vi "Handle Command.vi"(8 "error in":errorcluster, 10 "Change iSpkEn in":refnum<class "Change iSpk Signal.lvclass">, 11 "Object In":refnum<class>) -> (0 "error out":errorcluster, 1 "Command Successful?":bool, 2 "Change iSpkEn out":refnum<class "Change iSpk Signal.lvclass">, 3 "Object Out":refnum<class>)   [LabVIEW 2018, in "ePAS Library.lvlib" / "Change iSpk Signal.lvclass"]
doc: "Abstract method for accomplishing the execution of a command directed to an instrument object on the wire."
uses:
  Change iSpk Signal.lvclass
  Instrument/ePAS.lvclass
  C:/Users/Labview/Documents/exscalabar_server/reusable/Instrument/Instrument.lvclass
  Instrument/ePAS.lvclass/ePAS.ctl
  Change iSpk Signal.lvclass/Change iSpk Signal.ctl
  reusable/Instrument/Instrument.lvclass/Instrument.ctl
  reusable/Instrument/Read ExtCom.vi
  reusable/Instrument/Read Log Session.vi
  <vilib>/Utility/error.llb/Error Cluster From Error Code.vi
  <vilib>/rvi/errors/niLvFpgaAdjustHostInterfaceError.vi
  <userlib>/_Session Fwk/Session - Root.lvclass
  <vilib>/rvi/interface/nirviReadWriteControl/nirviReadWriteControl.xnode
  FPGA/R FPGA Ref.ctl
  FPGA Bitfiles/FPGAServer.lvbitx
  FPGA/Session/Exscalabar FPGA.lvclass
  ePAS Library.lvlib
  reusable/Session APIs/Session Log/System Log.lvclass
  NiFpgaLv.dll
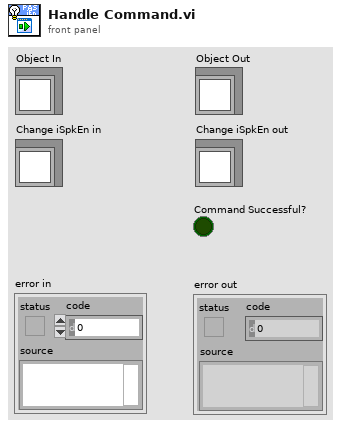
[diagram p1: front panel]
types:
  T1 = typedef "Session - Root.lvclass/Session Handle.ctl" = refnum<data-value>
  T2 = typedef "ePAS Library.lvlib/R FPGA Ref.ctl" = refnum<k20>
  T3 = cluster{"iSpkEn[0]":bool, "iSpkEn[1]":bool, "iSpkEn[2]":bool, "iSpkEn[3]":bool, "iSpkEn[4]":bool}
  T4 = cluster{"tag":string, "section":string, "data":variant}
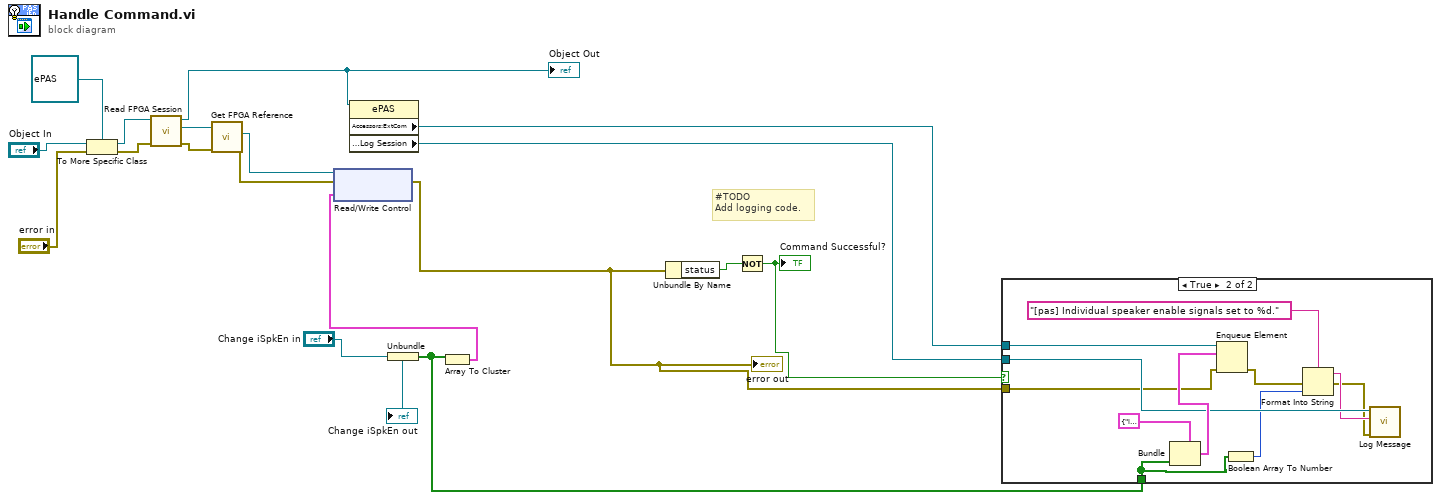
[diagram p0: block diagram]
diagram:
  # "#TODO\nAdd logging code."
  n1 = To More Specific Class(target class=refnum<class "ePAS.lvclass"> refnum ("ePAS"), reference="Object In", error in="error in") -> (specific class reference=w16:refnum<class "ePAS.lvclass">, error out=w15:errorcluster)
  n2 = call "Read FPGA Session.vi"("error in (no error)"=w15, "ePAS in"=w16) -> ("error out"=w11:errorcluster, "Session Handle"=w14:T1, "ePAS out"=w6:refnum<class "ePAS.lvclass">)  [unwired: 7 in]
  "Object Out" <- w6
  n3 = call "Get FPGA Reference.vi"("error in"=w11, "Session In"=w14) -> ("error out"=w9:errorcluster, "Ex FPGA Ref"=w13:T2)  [unwired: 7 in, 1 out]
  n4 = property class="ePAS"(reference=w6) -> ("Accessors:ExtCom"=w5:refnum<queue>, "Accessors:Log Session"=w3:T1)  [unwired: 1 in, 2 out]
  n5 = Unbundle("Change iSpkEn in") -> (w2:bool[])
  n6 = Array To Cluster(array=w2) -> (cluster=w8:T3)
  n7 = xnode "Read/Write Control"("FPGA VI Reference In"=w13, "error in"=w9, "iSpk Enable"=w8) -> ("error out"=w1:errorcluster)  [unwired: 1 out]
  "error out" <- w1
  n8 = Unbundle By Name(w1) -> ("status"=w7:bool)
  n9 = Not(x=w7) -> (.not. x?=w4:bool)
  "Command Successful?" <- w4
  n10 = case shown="True" w4 {
    tunnel: w5 -> [_ w29]
    tunnel: w2 -> [_ w22]
    tunnel: w3 -> [_ w26]
    tunnel: w1 -> [_ w21]
    frame False {
    }
    frame True {
      n11 = Bundle(cluster=T4 {"tag"="ienabled", "section"="pas.spk", "data"=variant} ("element"), "data"=w22) -> (w27:T4)  [unwired: 2 in]
      n12 = Enqueue Element(queue=w29, element=w27, error in (no error)=w21) -> (error out=w20:errorcluster)  [unwired: 1 in, 2 out]
      n13 = Boolean Array To Number(Boolean array=w22) -> (number=w24:u32)
      n14 = Format Into String(format string="[pas] Individual speaker enable signals set to %d.", error in=w20, w24) -> (resulting string=w23:string, error out=w19:errorcluster)  [unwired: 1 in]
      n15 = call "Log Message.vi"("error in"=w19, "MSG In"=w23, "session in"=w26) -> ()  [unwired: 7 in, 2 out]
    }
  }
  "Change iSpkEn out" <- "Change iSpkEn in"
